vi "test Add State.vi"(8 "error in (no error)":errorcluster, 11 "TestCase in":refnum<class "Routing and Faulting Scripting Unit Tests.lvclass">) -> (0 "error out":errorcluster, 3 "TestCase out":refnum<class "Routing and Faulting Scripting Unit Tests.lvclass">)   [LabVIEW 2017, in "Routing and Faulting Scripting Unit Tests.lvclass"]
uses:
  Routing and Faulting Scripting Unit Tests.lvclass
  Shared/Routing State.ctl
  Shared/Connection.ctl
  Routing and Faulting Scripting Unit Tests.lvclass/Routing and Faulting Scripting Unit Tests.ctl
  <vilib>/addons/_JKI Toolkits/VI Tester/TestCase.llb/TestCase.lvclass
  Routing and Faulting Scripting.lvlib
  Shared/Routing and Faulting Shared.lvlib
  C:/Program Files (x86)/National Instruments/LabVIEW 2017/vi.lib/addons/_JKI Toolkits/VI Tester/TestCase.llb/TestCase.lvclass
panel:
  in  "Save?":bool
  out "Output Filename":string
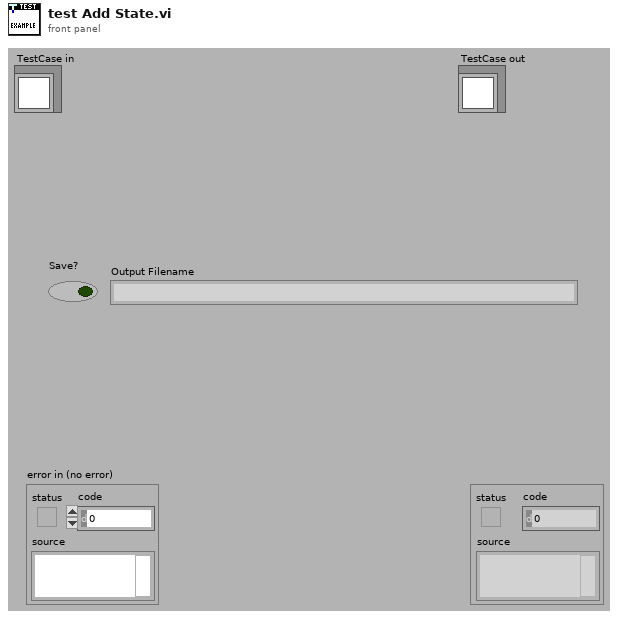
[diagram p1: front panel]
types:
  T1 = typedef "Routing and Faulting Shared.lvlib/Connection.ctl" = cluster{"Module":string, "Source":string, "Destination":string}
  T2 = typedef "Routing and Faulting Shared.lvlib/Routing State.ctl" = cluster{"Name":string, "Description":string, "Value":i32, "Connection List":T1[]}
  T3 = typedef "Custom Device API.lvlib/Custom Device Item Ref.ctl" = u64
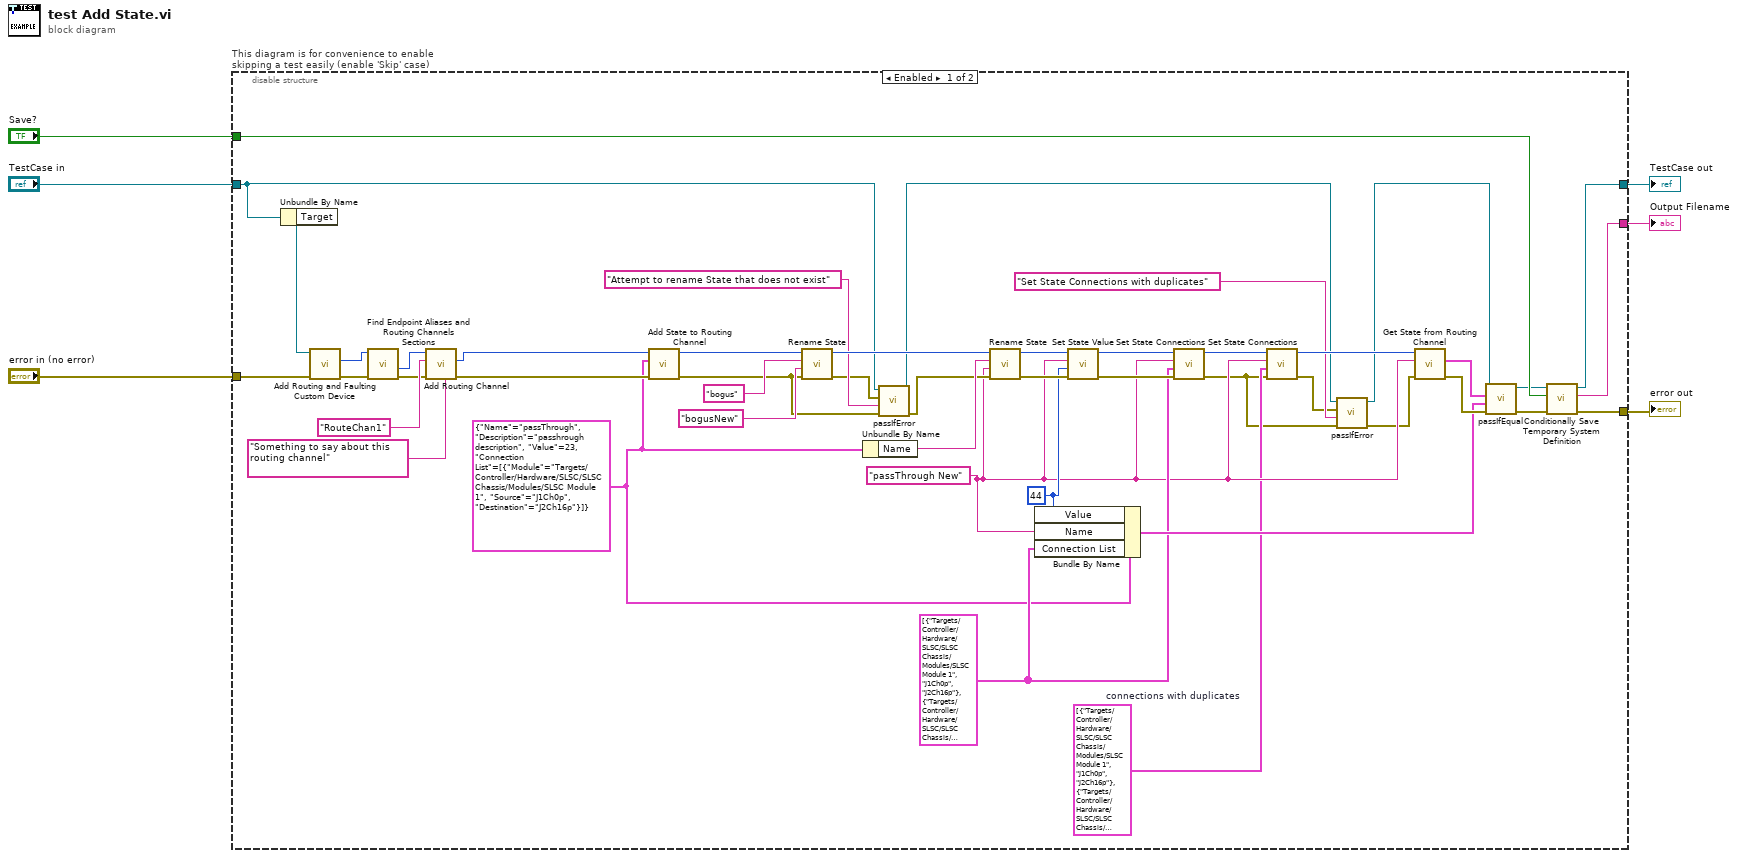
[diagram p0: block diagram]
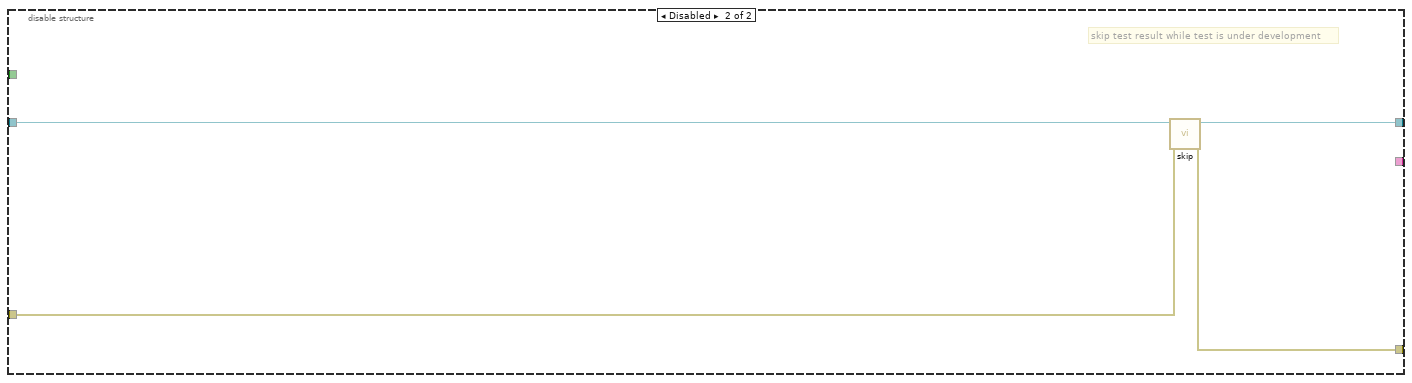
[diagram p2: hidden frame]
diagram:
  n1 = disable-structure "This diagram is for convenience to enable skipping a test easily (enable 'Skip' case)" shown="Enabled" {
    disable-tunnel: "TestCase in" -> [w27 w56]
    disable-tunnel: [w47 w54] -> w3
    disable-tunnel: [w51 w55] -> w5
    disable-tunnel: "error in (no error)" -> [w52 w53]
    disable-tunnel: [w50 _] -> w2
    disable-tunnel: "Save?" -> [w49 _]
    frame Enabled {
      w13 = T1[] [{"Module"="Targets/Controller/Hardware/SLSC/SLSC Chassis/Modules/SLSC Module 1", "Source"="J1Ch0p", "Destination"="J2Ch16p"}, {"Module"="Targets/Controller/Hardware/SLSC/SLSC Chassis/Modules/SLSC Module 1", "Source"="J1Ch0p", "Destination"="J2Ch16p"}]  # connections with duplicates
      w22 = T1[] [{"Module"="Targets/Controller/Hardware/SLSC/SLSC Chassis/Modules/SLSC Module 1", "Source"="J1Ch0p", "Destination"="J2Ch16p"}, {"Module"="Targets/Controller/Hardware/SLSC/SLSC Chassis/Modules/SLSC Module 1", "Source"="J1Ch0n", "Destination"="J2Ch16n"}] ("connection list")
      w37 = 44 ("New Value")
      w14 = "passThrough New" ("New State")
      w17 = T2 {"Name"="passThrough", "Description"="passhrough description", "Value"=23, "Connection List"=[{"Module"="Targets/Controller/Hardware/SLSC/SLSC Chassis/Modules/SLSC Module 1", "Source"="J1Ch0p", "Destination"="J2Ch16p"}]} ("Routing State")
      n2 = Unbundle By Name(w27) -> ("Target"=w48:refnum<k24>)
      n3 = call "Add Routing and Faulting Custom Device.vi"("error in (no error)"=w52, "Target in"=w48) -> ("error out"=w46:errorcluster, "Routing and Faulting Custom Device Ref"=w20:T3)  [unwired: 7 in, 1 out]
      n4 = call "Find Endpoint Aliases and Routing Channels Sections.vi"("error in (no error)"=w46, "Routing and Faulting Custom Device Ref in"=w20) -> ("error out"=w21:errorcluster, "Routing Channels Ref"=w19:T3)  [unwired: 6 in, 2 out]
      n5 = call "Add Routing Channel.vi"("Description"="Something to say about this routing channel", "error in (no error)"=w21, "Channel Name"="RouteChan1", "Routing Channels Ref in"=w19) -> ("error out"=w42:errorcluster, "Channel Ref"=w41:T3)  [unwired: 5 in, 1 out]
      n6 = call "Add State to Routing Channel.vi"("error in (no error)"=w42, "State and Connections"=w17, "Channel Ref in"=w41) -> ("error out"=w31:errorcluster, "Channel Ref out"=w35:T3)  [unwired: 7 in]
      n7 = call "Rename State.vi"("error in (no error)"=w31, "New State"="bogusNew" ("State"), "State"="bogus", "Channel Ref in"=w35) -> ("error out"=w29:errorcluster, "Channel Ref out"=w34:T3)  [unwired: 6 in]
      n8 = Unbundle By Name(w17) -> ("Name"=w40:string)
      n9 = call-dynamic "passIfError.vi"("error in (no error)"=w31, "task (\"\")"="Attempt to rename State that does not exist" ("custom report message (\"\")"), "error"=w29, "TestCase in"=w27) -> ("error out"=w28:errorcluster, "TestCase out"=w10:refnum<class "Routing and Faulting Scripting Unit Tests.lvclass">)  [unwired: 6 in]
      n10 = call "Rename State.vi"("error in (no error)"=w28, "New State"=w14, "State"=w40, "Channel Ref in"=w34) -> ("error out"=w38:errorcluster, "Channel Ref out"=w39:T3)  [unwired: 6 in]
      n11 = Bundle By Name(cluster=w17, "Value"=w37, "Name"=w14, "Connection List"=w22) -> (w25:T2)
      n12 = call "Set State Value.vi"("error in (no error)"=w38, "New Value"=w37, "State"=w14, "Channel Ref in"=w39) -> ("error out"=w24:errorcluster, "Channel Ref out"=w23:T3)  [unwired: 6 in]
      n13 = call "Set State Connections.vi"("error in (no error)"=w24, "Connection List"=w22, "State"=w14, "Channel Ref in"=w23) -> ("error out"=w12:errorcluster, "Channel Ref out"=w16:T3)  [unwired: 6 in]
      n14 = call "Set State Connections.vi"("error in (no error)"=w12, "Connection List"=w13, "State"=w14, "Channel Ref in"=w16) -> ("error out"=w8:errorcluster, "Channel Ref out"=w15:T3)  [unwired: 6 in]
      n15 = call-dynamic "passIfError.vi"("error in (no error)"=w12, "task (\"\")"="Set State Connections with duplicates" ("task (\"\")"), "error"=w8, "TestCase in"=w10) -> ("error out"=w7:errorcluster, "TestCase out"=w9:refnum<class "Routing and Faulting Scripting Unit Tests.lvclass">)  [unwired: 6 in]
      n16 = call "Get State from Routing Channel.vi"("error in (no error)"=w7, "State"=w14, "Channel Ref in"=w15) -> ("error out"=w36:errorcluster, "State and Connections"=w26:T2)  [unwired: 6 in, 1 out]
      n17 = call-dynamic "passIfEqual.vi"("error in (no error)"=w36, "y"=w25, "x"=w26, "TestCase in"=w9) -> ("error out"=w45:errorcluster, "TestCase out"=w44:refnum<class "Routing and Faulting Scripting Unit Tests.lvclass">)  [unwired: 6 in]
      n18 = call "Conditionally Save Temporary System Definition.vi"("error in (no error)"=w45, "Save?"=w49, "Test Case"=w44) -> ("error out"=w51:errorcluster, "filename"=w50:string, "Test Case"=w47:refnum<class "Routing and Faulting Scripting Unit Tests.lvclass">)  [unwired: 6 in]
    }
    frame Disabled {
      # "skip test result while test is under development"
      n19 = call <vilib>:"skip.vi"("error in (no error)"=w53, "TestCase in"=w56) -> ("error out"=w55:errorcluster, "TestCase out"=w54:refnum<class "Routing and Faulting Scripting Unit Tests.lvclass">)  [unwired: 8 in]
    }
  }
  "error out" <- w5
  "TestCase out" <- w3
  "Output Filename" <- w2
